vi "SaccadeAnalyser - Calc 3D Angular Derivative.vi"(1 "Sample Rate (Hz)":dbl=500.0 format="%#_13g", 2 "RPY Position":dbl[][](array[numeric])) -> (0 "RPY Velocity":dbl[][](array[numeric]))   [LabVIEW 2016]
uses:
  <vilib>/Analysis/NI_AALPro.lvlib
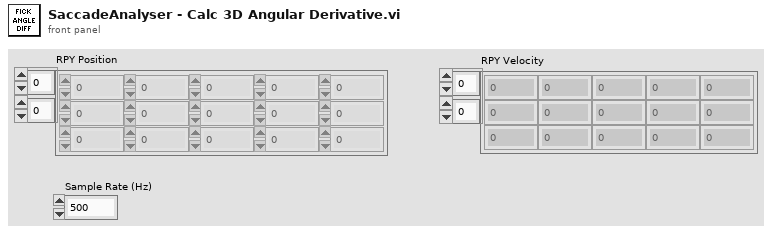
[diagram p1: front panel]
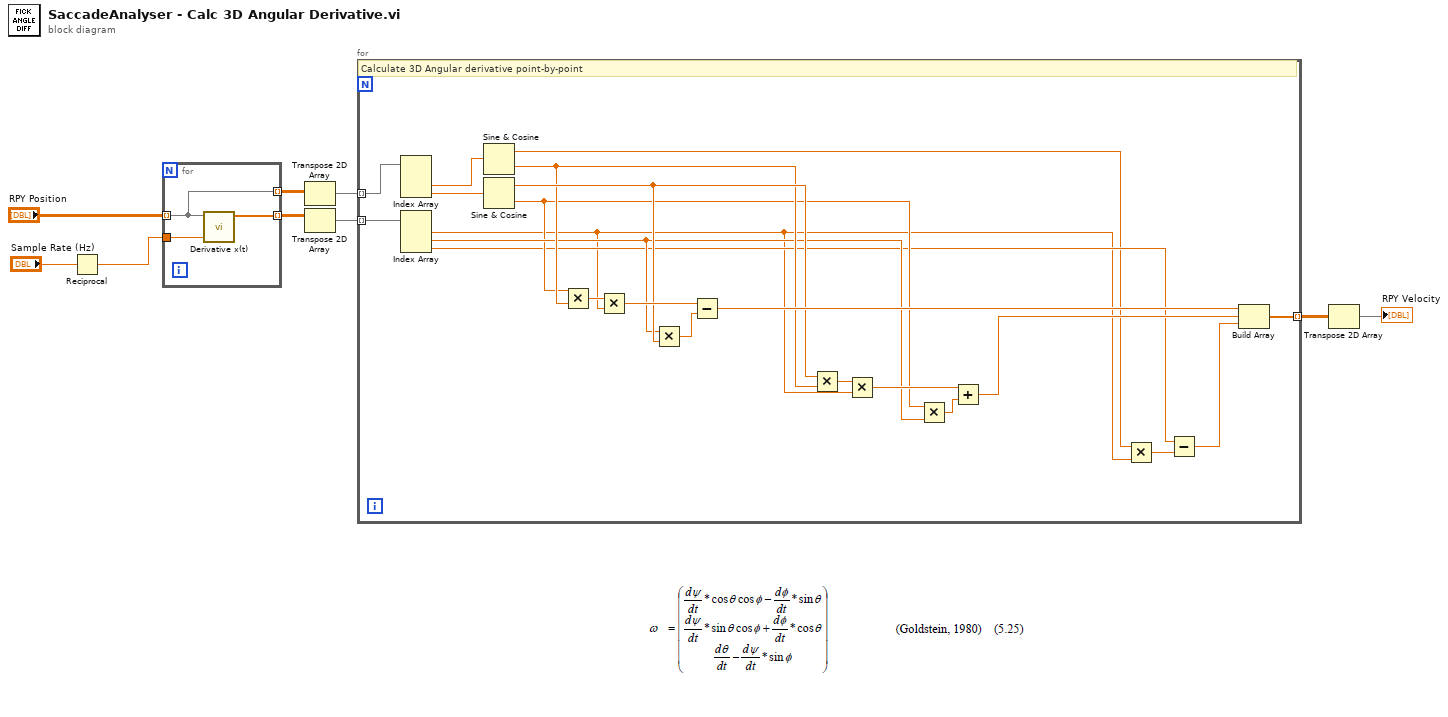
[diagram p0: block diagram]
diagram:
  n1 = Reciprocal(x="Sample Rate (Hz)") -> (1/x=w1:dbl)
  n2 = for {
    tunnel: "RPY Position" -> [w10] mode=indexing
    tunnel: [w12] -> w6 mode=indexing
    tunnel: w1 -> [w11]
    tunnel: [w10] -> w7 mode=indexing
    n3 = call <vilib>:"Derivative x(t).vi"("dt"=w11, "X"=w10) -> ("dX/dt"=w12:dbl[])  [unwired: 8 in, 1 out]
  }
  n4 = Transpose 2D Array(2D array=w7) -> (transposed array=w5:dbl[][])
  n5 = Transpose 2D Array(2D array=w6) -> (transposed array=w4:dbl[][])
  n6 = for {
    tunnel: w5 -> [w34] mode=indexing
    tunnel: w4 -> [w33] mode=indexing
    tunnel: [w26] -> w3 mode=indexing
    # "Calculate 3D Angular derivative point-by-point"
    n7 = Index Array(array=w34) -> (element #2=w31:dbl, element #3=w32:dbl)  [unwired: 3 in, 1 out]
    n8 = Index Array(array=w33) -> (element #1=w14:dbl, element #2=w19:dbl, element #3=w17:dbl)  [unwired: 3 in]
    n9 = Sine & Cosine(0:w31) -> (1:w15:dbl, 2:w24:dbl)
    n10 = Sine & Cosine(0:w32) -> (1:w25:dbl, 2:w18:dbl)
    n11 = Multiply(x=w18, y=w24) -> (x*y=w30:dbl)
    n12 = Multiply(x=w30, y=w14) -> (x*y=w29:dbl)
    n13 = Multiply(x=w19, y=w25) -> (x*y=w28:dbl)
    n14 = Subtract(x=w29, y=w28) -> (x-y=w27:dbl)
    n15 = Multiply(x=w25, y=w24) -> (x*y=w23:dbl)
    n16 = Multiply(x=w23, y=w14) -> (x*y=w22:dbl)
    n17 = Multiply(x=w18, y=w19) -> (x*y=w21:dbl)
    n18 = Add(x=w22, y=w21) -> (x+y=w20:dbl)
    n19 = Multiply(x=w15, y=w14) -> (x*y=w16:dbl)
    n20 = Subtract(x=w17, y=w16) -> (x-y=w13:dbl)
    n21 = Build Array(w27, w20, w13) -> (w26:dbl[])
  }
  n22 = Transpose 2D Array(2D array=w3) -> (transposed array=→"RPY Velocity":dbl[][])
